vi "Init.vi"(8 "error in (no error)":errorcluster, 9 "Config File Path":path=path "", 10 "Name":string, 11 "Mock Error Handler In":refnum<class "Mock Error Handler.lvclass">) -> (0 "error out":errorcluster, 3 "Mock Error Handler Out":refnum<class "Mock Error Handler.lvclass">)   [LabVIEW 2020, in "Mock Error Handler.lvclass"]
doc: "Initializes the process and creates necessary references. Anything initialized here is released in the Clear.vi method."
uses:
  Mock Error Handler.lvclass
  Private/Error Message Data.ctl
  Mock Error Handler.lvclass/Mock Error Handler.ctl
  Framework/Base/Base.lvclass
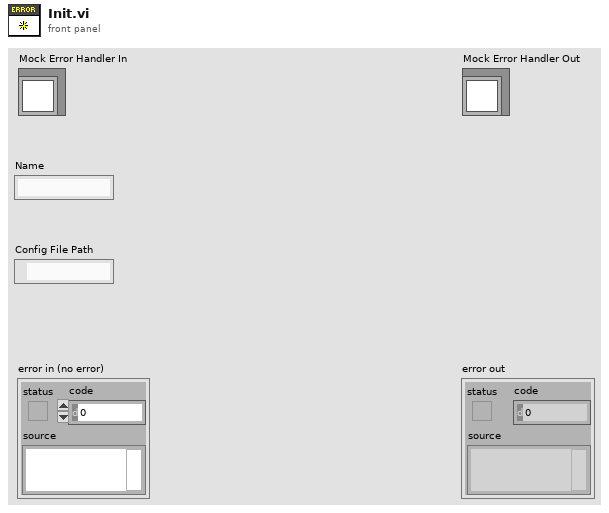
[diagram p1: front panel]
types:
  T1 = typedef "Mock Error Handler.lvclass/Error Message Data.ctl" = cluster{"Location":string, "Error":errorcluster}
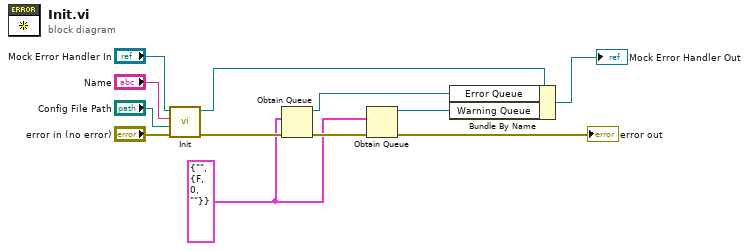
[diagram p0: block diagram]
diagram:
  w2 = T1 {"Location"="", "Error"={"status"=FALSE, "code"=0, "source"=""}} ("Error Message Data")
  n1 = call-parent "Init.vi"("error in (no error)"="error in (no error)", "Config File Path"="Config File Path", "Name"="Name", "Base In"="Mock Error Handler In") -> ("error out"=w6:errorcluster, "Base Out"=w8:refnum<class "Mock Error Handler.lvclass">)  [unwired: 6 in]
  n2 = Obtain Queue(element data type=w2, error in (no error)=w6) -> (queue out=w5:refnum<queue>, error out=w4:errorcluster)  [unwired: 3 in, 1 out]
  n3 = Obtain Queue(element data type=w2, error in (no error)=w4) -> (queue out=w1:refnum<queue>, error out=→"error out":errorcluster)  [unwired: 3 in, 1 out]
  n4 = Bundle By Name(cluster=w8, "Error Queue"=w5, "Warning Queue"=w1) -> (→"Mock Error Handler Out":refnum<class "Mock Error Handler.lvclass">)
